vi "GetPos.vi"(0 "System no.":i32=1 min=1 step=1, 5 "error in":errorcluster, 12 "Stop refnum":refnum<vi>) -> (15 "Position":dbl[](array[numeric]) format="%.6f", 19 "error out":errorcluster)   [LabVIEW 2014]
doc: "This VI is runs in a loop until the stop button is pressed, the stop reference is TRUE or an error occures. It lets the operator set the velocity, move the connected axes to relative, absolute or to the home position, and reads the current position continuosly. The diagram shows how to combine the driver and support VIs for these tasks. Use the Help?Show Context Help menu sequence in the LabVIEW environment to display the Context Help window with the VI and control/indicator descriptions.\nRun \" XXXX_Configuration_Setup.vi\" (with XXXX being the PI product number of your system) prior to running this VI. \n\nValid for: C-843, C-843.PM, C-865, C-866, Mercury"
uses:
  C:/Users/Public/PI/GCSMergedLabVIEW/Low Level/General command.llb/Global2 (Array).vi
panel:
  in  "stop":bool
  out "Conn. Axes":string[](array[string])
  # "Command move:"
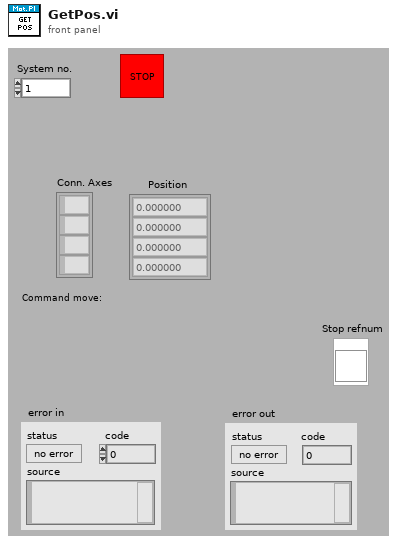
[diagram p1: front panel]
types:
  T1 = typedef "Controller names.ctl" = enum16{"None", "Analog", "C-702", "C-843", "C-843.PM", "C-844", "C-848", "C-865", "C-866", "C-867", "C-880", "C-884", "E-516", "E-517", "E-709", "E-710", "E-712", "E-725", "E-753", "E-755", "E-761", "E-816", "E-861", "E-870", "F-206", "HydraPollux", "M-840", "M-850", "M-8X0", "Mercury", "Mercury_GCS"}
  T2 = cluster{"Conn. axes":string[], "Controller name":T1}[]
  T3 = cluster{"Conn. axes":string[], "Controller name":T1}
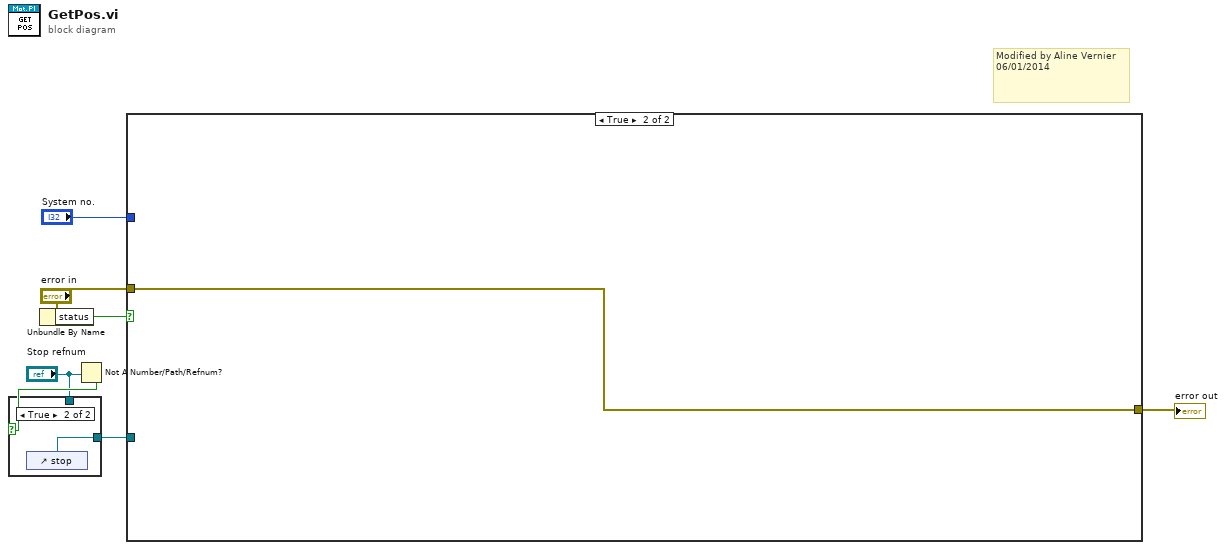
[diagram p0: block diagram]
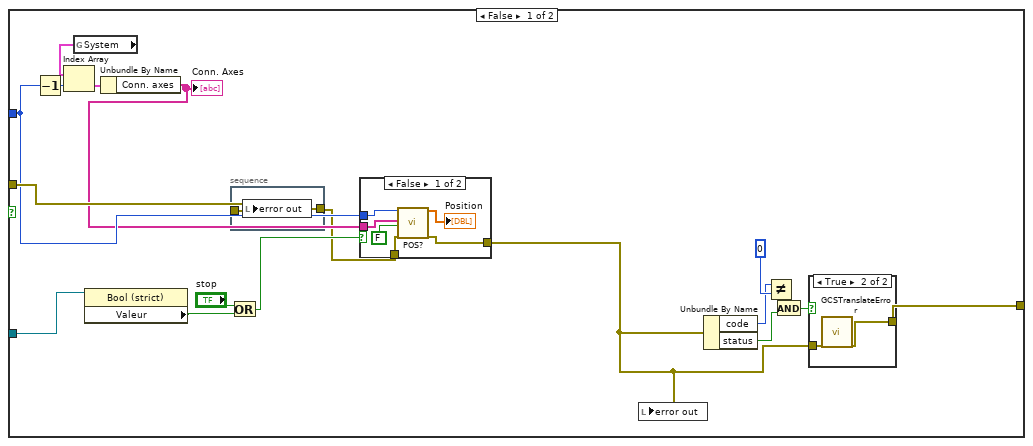
[diagram p3: hidden frame]
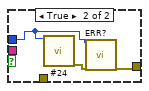
[diagram p5: hidden frame]
diagram:
  # "Modified by Aline Vernier\n06/01/2014"
  n1 = Unbundle By Name("error in") -> ("status"=w6:bool)
  n2 = Not A Number/Path/Refnum?(number/path/refnum="Stop refnum") -> (NaN/Path/Refnum?=w3:bool)
  n3 = case shown="True" w3 {
    tunnel: [w8 w9] -> w2
    tunnel: "Stop refnum" -> [w8 _]
    frame False {
    }
    frame True {
      n4 = control-ref of="stop"() -> (w9:refnum<vi>)
    }
  }
  n5 = case shown="True" w6 {
    tunnel: [w27 w40] -> w5
    tunnel: "error in" -> [w26 w40]
    tunnel: "System no." -> [w23 _]
    tunnel: w2 -> [w25 _]
    frame False {
      n6 = Decrement(x=w23) -> (x-1=w22:i32)
      n7 = global read "Global2 (Array).vi" "System"() -> (w21:T2)
      n8 = Index Array(array=w21, index=w22) -> (element=w20:T3)
      n9 = property class="Bool (strict)"(reference=w25) -> ("Valeur"=w18:bool)  [unwired: 1 in, 2 out]
      n10 = Unbundle By Name(w20) -> ("Conn. axes"=w14:string[])
      "Conn. Axes" <- w14
      n11 = Or(x="stop", y=w18) -> (x .or. y?=w15:bool)
      n12 = stacked-sequence {
        tunnel: w26 -> [w39]
        tunnel: [w39] -> w11
        frame #0 {
          n13 = local write "error out"(w39) -> ()
        }
      }
      n14 = case shown="False" w15 {
        tunnel: w23 -> [w31 w38]
        tunnel: [w34 w36] -> w10
        tunnel: w14 -> [w32 _]
        tunnel: w11 -> [w30 _]
        frame False {
          n15 = call "POS?.vi"("System no."=w31, "Axes to query"=w32, "All axes?"=FALSE, "error in"=w30) -> ("Position"=→"Position":dbl[], "error out"=w34:errorcluster)  [unwired: 14 in]
        }
        frame True {
          n16 = call "#24.vi"("System no."=w38) -> ("error out"=w37:errorcluster)  [unwired: 18 in]
          n17 = call "ERR?.vi"("System no."=w38, "error in"=w37) -> ("error out"=w36:errorcluster)  [unwired: 16 in, 1 out]
        }
      }
      n18 = local write "error out"(w10) -> ()
      n19 = Unbundle By Name(w10) -> ("code"=w13:i32, "status"=w12:bool)
      n20 = Not Equal?(x=w13, y=0 ("code")) -> (x != y?=w17:bool)
      n21 = And(x=w17, y=w12) -> (x .and. y?=w16:bool)
      n22 = case shown="True" w16 {
        tunnel: [_ w29] -> w27
        tunnel: w10 -> [_ w28]
        frame False {
        }
        frame True {
          n23 = call "GCSTranslateError.vi"("error in"=w28) -> ("error out"=w29:errorcluster)  [unwired: 16 in, 2 out]
        }
      }
    }
    frame True {
    }
  }
  "error out" <- w5
